vi "DAQmx Create Channel (CI-Velocity-Linear).vi"(0 "task in":refnum<k21>, 1 "maximum value":dbl=1.0, 2 "minimum value":dbl, 5 "counter":tag, 6 "decoding type":i32(ring)=10092 items=["X1"=10090, "X2"=10091, "X4"=10092, "Two Pulse Counting"=10313], 7 "name to assign":string, 9 "units":i32(ring)=15959 items=["in/s"=15960, "m/s"=15959, "From Custom Scale"=10065], 11 "error in":errorcluster, 12 "custom scale name":tag, 13 "distance per pulse":dbl=0.001) -> (4 "task out":refnum<k21>, 15 "error out":errorcluster)   [LabVIEW 2020]
doc: "Creates a channel that uses a linear encoder to measure linear velocity. With the exception of devices that support multi-counter tasks, you can create only one counter input channel at a time with this VI because a task can contain only one counter input channel. To read from multiple counters simultaneously, use a separate task for each counter. Connect the input signal to the default input terminal of the counter unless you select a different input terminal."
uses:
  nilvaiu.dll
panel:
  # "input limits"
  # "encoder info"
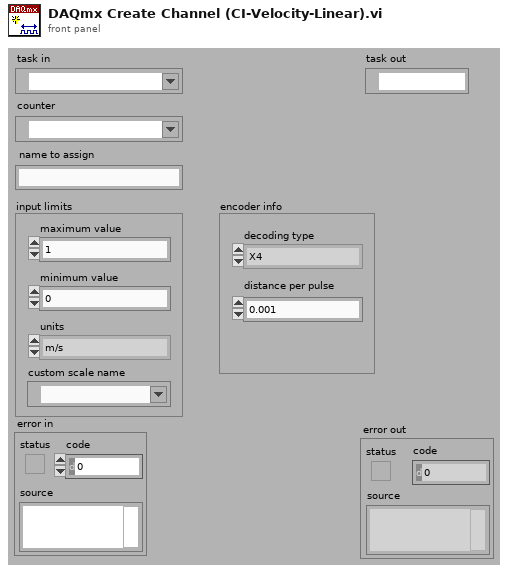
[diagram p1: front panel]
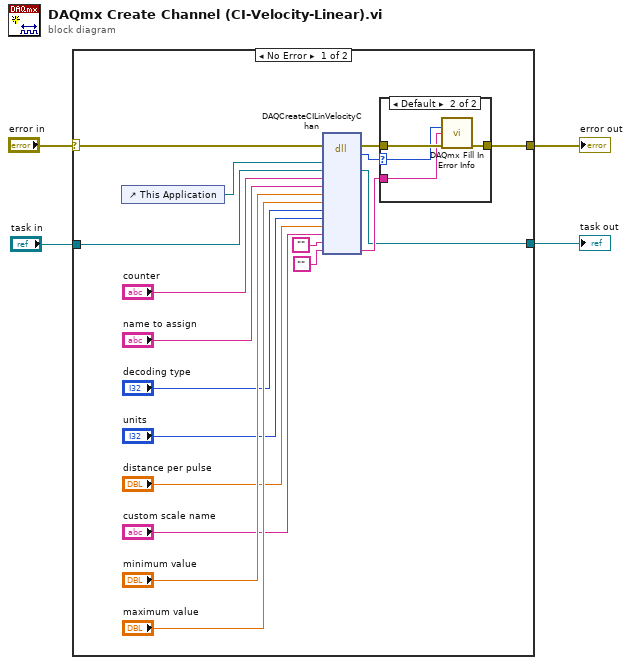
[diagram p0: block diagram]
diagram:
  n1 = case shown="No Error" "error in" {
    selector: "error in" -> [w6 w29]
    tunnel: [w9 w29] -> w4
    tunnel: [w8 w28] -> w3
    tunnel: "task in" -> [w7 w28]
    frame No Error {
      n2 = control-ref of="This Application"() -> (w19:refnum<vi>)
      n3 = dll-call lib="nilvaiu.*" fn="DAQCreateCILinVelocityChan"(error in=w6, "lvAppRef"=w19, "refObjPtr"=w7, "counter"="counter", "channelNameIn"="name to assign", "minVal"="minimum value", "maxVal"="maximum value", "decodingType"="decoding type", "units"="units", "distsPerPulse"="distance per pulse", "customScaleName"="custom scale name", "channelNamesOut"="", "extendedErrorInfo"="") -> (error out=w22:errorcluster, "return type"=w21:i32, "refObjPtr"=w8:refnum<k21>, "extendedErrorInfo"=w20:string)  [unwired: 12 in, 1 out]
      n4 = case shown="Default" w21 {
        selector: w21 -> [_ w25]
        tunnel: w22 -> [w23 w27]
        tunnel: [w23 w26] -> w9
        tunnel: w20 -> [_ w24]
        frame 0 {
        }
        frame Default {
          n5 = call "DAQmx Fill In Error Info.vi"("status code"=w25, "extended error info"=w24, "error in"=w27) -> ("error out"=w26:errorcluster)  [unwired: 1 in, 11 out]
        }
      }
    }
    frame Error {
    }
  }
  "error out" <- w4
  "task out" <- w3
